vi "dsdll_config.vi"(8 "error in":errorcluster, 9 "capture thread idle [ms]":i32 min=0 max=500, 10 "capture thread priority":i32(ring)=-256 items=["don't modify"=-256, "IDLE"=-15, "LOWEST"=-2, "BELOW NORMAL"=-1, "NORMAL"=0, "ABOVE NORMAL"=1, "HIGHEST"=2, "TIME CRITICAL"=15], 11 "dsdll instance in":T1={"dsdll path"=path "E:/LVprog/DirectSoundDLL/dsdll.dll", "dsdll handle"=[], "output devices"=[], "capture devices"=[]}) -> (0 "error out":errorcluster, 3 "dsdll instance out":T1)   [LabVIEW 2013, in "dsdll.lvlib"]
doc: "Call this to configurate opened DSDLL instance.\n\nOption 'capture thread idle' sets capture buffer read interval in miliseconds. It should be set in range 1 to 500 ms. Lower values should be used to decrease capture latency. Default is 10 ms.\n\nOption 'capture thread priority' sets priority of the capture thread. It is usually ABOVE NORMAL but in case of underflows it may be increased. The values passed to the function are directly passed to SetThreadPriority() WINAPI so look for details at MSDN."
uses:
  dsdll.lvlib
  dsdll_instance.ctl
  dsdll_device_record.ctl
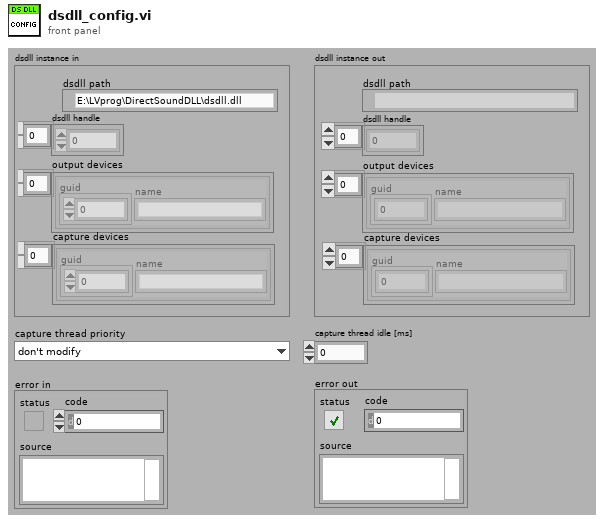
[diagram p1: front panel]
types:
  T1 = typedef "dsdll.lvlib/dsdll_instance.ctl" = cluster{"dsdll path":path, "dsdll handle":u8[], "output devices":T2[], "capture devices":T2[]}
  T2 = typedef "dsdll.lvlib/dsdll_device_record.ctl" = cluster{"guid":u8[], "name":string}
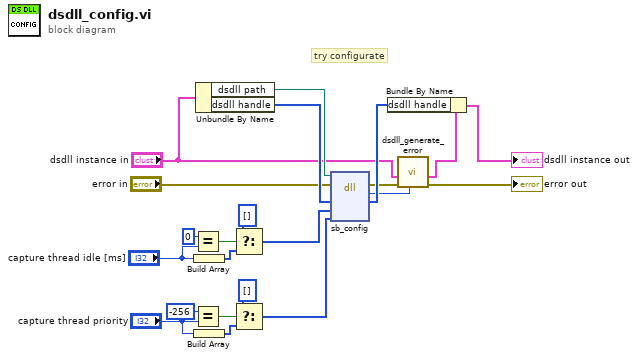
[diagram p0: block diagram]
diagram:
  # "try configurate"
  n1 = Equal?(x=0, y="capture thread idle [ms]") -> (x = y?=w8:bool)
  n2 = Equal?(x=-256, y="capture thread priority") -> (x = y?=w17:bool)
  n3 = Build Array("capture thread idle [ms]") -> (w10:i32[])
  n4 = Build Array("capture thread priority") -> (w15:i32[])
  n5 = Unbundle By Name("dsdll instance in") -> ("dsdll path"=w21:path, "dsdll handle"=w20:u8[])
  n6 = Select(t=i32[] [], s=w8, f=w10) -> (s? t:f=w7:i32[])
  n7 = Select(t=i32[] [], s=w17, f=w15) -> (s? t:f=w12:i32[])
  n8 = dll-call lib="dsdll.dll" fn="sb_config" ("sb_get_handle_size()")(path in=w21, error in="error in", "handle"=w20, "capt_idle"=w7, "capt_prior"=w12) -> (error out=w5:errorcluster, "error"=w3:i32, "handle"=w19:u8[])  [unwired: 3 in, 1 out]
  n9 = call "dsdll_generate_error.vi"("error code"=w3, "error in"=w5, "dsdll instance in"="dsdll instance in") -> ("error out"=→"error out":errorcluster, "dsdll instance out"=w1:T1)  [unwired: 6 in, 1 out]
  n10 = Bundle By Name(cluster=w1, "dsdll handle"=w19) -> (→"dsdll instance out":T1)
